vi "Destruction.vi"(8 "error in (no error)":errorcluster, 11 "RT FIFO I64 Notifier in":refnum<class "RT FIFO I64 Notifier.lvclass">) -> (0 "error out":errorcluster, 3 "RT FIFO I64 Notifier out":refnum<class "RT FIFO I64 Notifier.lvclass">)   [LabVIEW 2024, in "RT FIFO I64 Notifier.lvclass"]
uses:
  RT FIFO I64 Notifier.lvclass
  RT FIFO I64 Notifier.lvclass/RT FIFO I64 Notifier.ctl
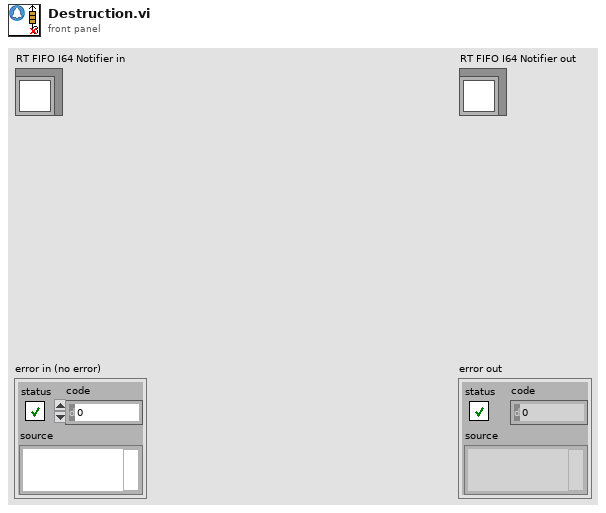
[diagram p1: front panel]
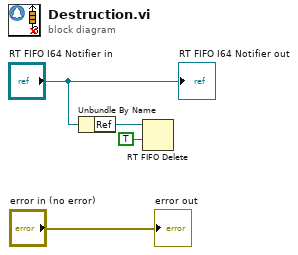
[diagram p0: block diagram]
diagram:
  n1 = Unbundle By Name("RT FIFO I64 Notifier in") -> ("Ref"=w2:refnum<k33>)
  n2 = RT FIFO Delete(0:w2, 2:TRUE ("force destroy? (F)")) -> ()  [unwired: 1 in, 1 out]
  "error out" <- "error in (no error)"
  "RT FIFO I64 Notifier out" <- "RT FIFO I64 Notifier in"
